vi "Remove Connection from List (data structure)vi.vi"(8 "error in (no error)":errorcluster, 10 "Connection":T1, 11 "connection list in":T1[](array[typedef])) -> (0 "error out":errorcluster, 1 "removed":bool, 3 "connection list out":T1[](array[typedef]))   [LabVIEW 2017, in "Switch Scripting.lvlib"]
uses:
  Switch Scripting.lvlib
  Connection.ctl
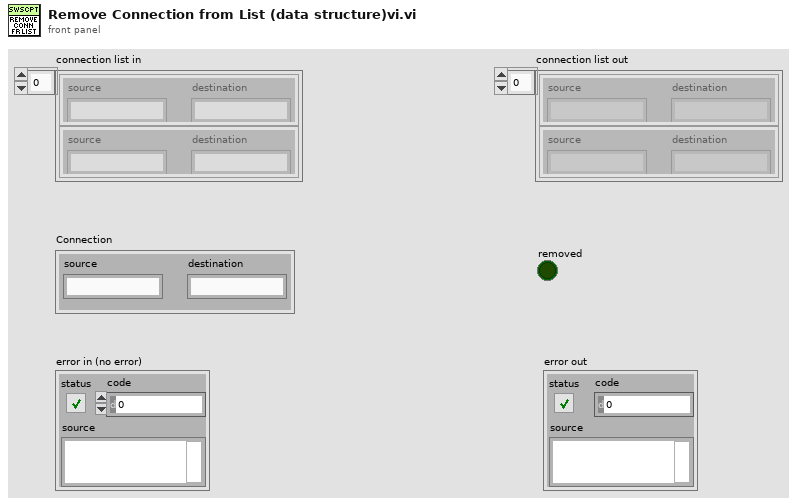
[diagram p1: front panel]
types:
  T1 = typedef "Switch Scripting.lvlib/Connection.ctl" = cluster{"source":string, "destination":string}
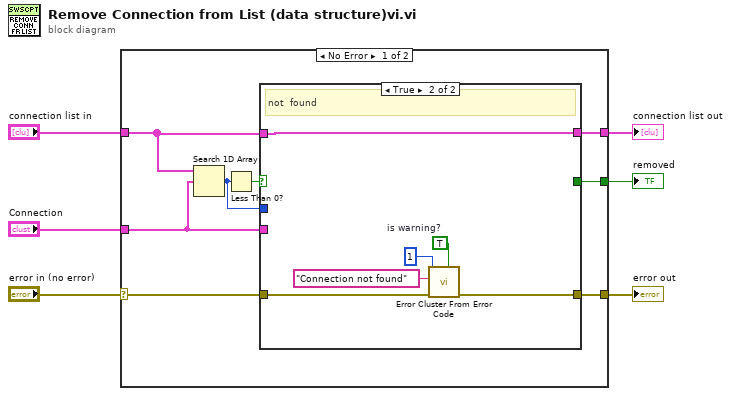
[diagram p0: block diagram]
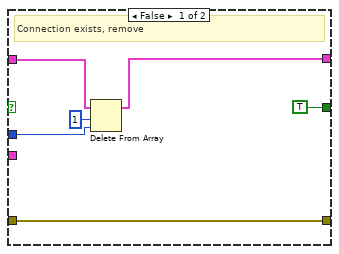
[diagram p2: hidden frame]
diagram:
  n1 = case shown="No Error" "error in (no error)" {
    selector: "error in (no error)" -> [w14 w28]
    tunnel: [w13 w28] -> w6
    tunnel: [w8 w27] -> w5
    tunnel: "connection list in" -> [w9 w27]
    tunnel: "Connection" -> [w10 _]
    tunnel: [w11 _] -> w1
    frame No Error {
      n2 = Search 1D Array(1D array=w9, element=w10) -> (index of element=w7:i32)  [unwired: 1 in]
      n3 = Less Than 0?(x=w7) -> (x < 0?=w12:bool)
      n4 = case shown="True" w12 {
        tunnel: w14 -> [w16 w21]
        tunnel: [w16 w23] -> w13
        tunnel: [TRUE _] -> w11
        tunnel: w9 -> [w19 w22]
        tunnel: w10 -> [_ _]
        tunnel: [w15 w22] -> w8
        tunnel: w7 -> [w17 _]
        frame False {
          # "Connection exists, remove"
          n5 = Delete From Array(array=w19, length=1, index=w17) -> (array with subset deleted=w15:T1[])  [unwired: 1 out]
        }
        frame True {
          w25 = TRUE  # is warning?
          # "not  found"
          n6 = call <vilib>:"Error Cluster From Error Code.vi"("is warning? (False)"=w25, "error in (no error)"=w21, "error message (\"\")"="Connection not found" ("error message (\"\")"), "error code (0)"=1) -> ("error out"=w23:errorcluster)  [unwired: 5 in]
        }
      }
    }
    frame Error {
    }
  }
  "error out" <- w6
  "connection list out" <- w5
  "removed" <- w1
